vi "Untitled 3 (SubVI).vi"(6 "V Range":dbl, 7 "Initial V":dbl, 9 "Numeric 3":i32, 10 "Numeric in":i32, 11 "Number of samples":i32=10) -> (1 "mean":dbl, 2 "Numeric out":dbl, 3 "Voltage":dbl format="%0.2f", 4 "Current":dbl format="%0.2f")   [LabVIEW 2016]
uses:
  <vilib>/Analysis/baseanly.llb/Mean (DBL).vi
  <vilib>/Analysis/NI_AALBase.lvlib
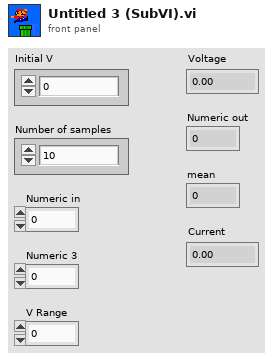
[diagram p1: front panel]
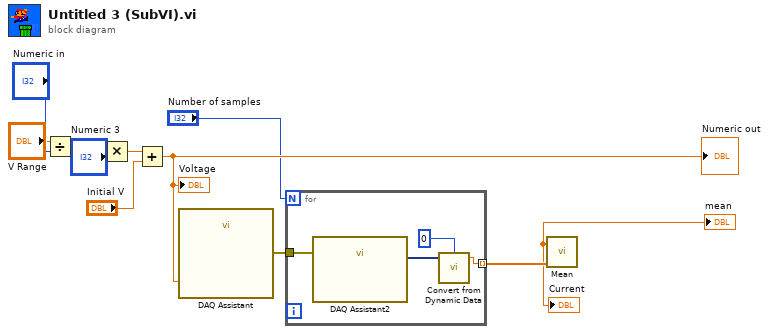
[diagram p0: block diagram]
diagram:
  n1 = Divide(x="V Range", y="Numeric in") -> (x/y=w4:dbl)
  n2 = Multiply(x=w4, y="Numeric 3") -> (x*y=w10:dbl)
  n3 = Add(x=w10, y="Initial V") -> (x+y=w11:dbl)
  "Voltage" <- w11
  "Numeric out" <- w11
  n4 = call "DAQ Assistant"("data"=w11) -> ("error out"=w3:errorcluster)  [unwired: 17 in, 1 out]
  n5 = for {
    N: "Number of samples" -> [_]
    tunnel: w3 -> [w15]
    tunnel: [w14] -> w2 mode=indexing
    n6 = call "DAQ Assistant2"("error in"=w15) -> ("data"=w13:dynamicdata)  [unwired: 16 in, 2 out]
    n7 = call "Convert from Dynamic Data"("Dynamic Data Type"=w13, "Channel"=0) -> ("Scalar"=w14:dbl)  [unwired: 2 in]
  }
  n8 = call-poly <vilib>:"Mean.vi"("X"=w2) -> ("mean"=→"Current" →"mean":dbl)  [unwired: 1 out]
